vi "Driverstation.vi"   [LabVIEW 2012]
uses:
  Robot Global Data.vi
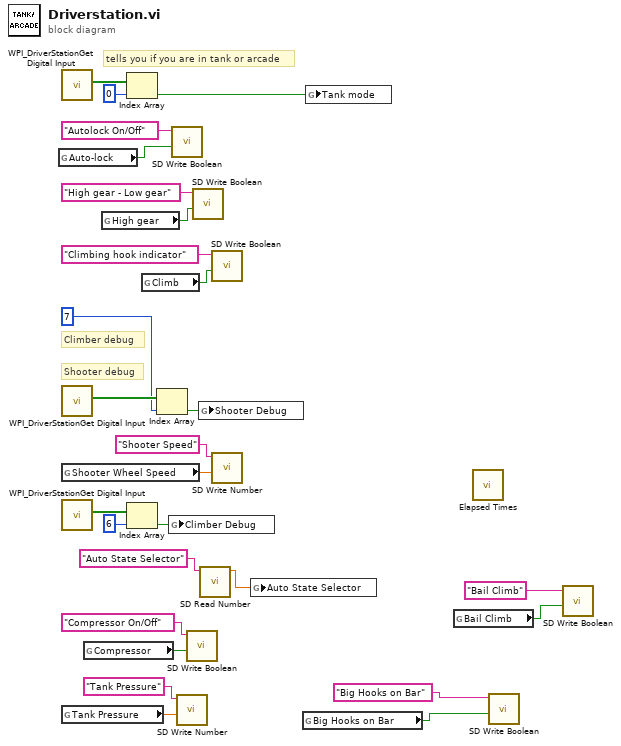
[diagram p0: block diagram]
diagram:
  # "Climber debug"
  # "Shooter debug"
  # "tells you if you are in tank or arcade"
  n1 = global read "Robot Global Data.vi" "Auto-lock"() -> (w5:bool)
  n2 = call <vilib>:"WPI_DriverStationGet Digital Input.vi"() -> ("Driver Station Digital Input (1-8)"=w27:bool[])  [unwired: 11 in]
  n3 = call <vilib>:"WPI_DriverStationGet Digital Input.vi"() -> ("Driver Station Digital Input (1-8)"=w24:bool[])  [unwired: 11 in]
  n4 = global read "Robot Global Data.vi" "Shooter Wheel Speed"() -> (w11:dbl)
  n5 = call <vilib>:"WPI_DriverStationGet Digital Input.vi"() -> ("Driver Station Digital Input (1-8)"=w20:bool[])  [unwired: 11 in]
  n6 = global read "Robot Global Data.vi" "Tank Pressure"() -> (w10:dbl)
  n7 = global read "Robot Global Data.vi" "Compressor"() -> (w9:bool)
  n8 = global read "Robot Global Data.vi" "High gear"() -> (w18:bool)
  n9 = Index Array(array=w27, index=0) -> (element=w25:bool)
  n10 = Index Array(array=w20, index=6) -> (element=w19:bool)
  n11 = global read "Robot Global Data.vi" "Climb"() -> (w15:bool)
  n12 = Index Array(array=w24, index=7) -> (element=w22:bool)
  n13 = global write "Robot Global Data.vi" "Climber Debug"(w19) -> ()
  n14 = call <vilib>:"SD Write Boolean.vi"("Boolean"=w5, "Name"="Autolock On/Off") -> ()  [unwired: 8 in, 2 out]
  n15 = call <vilib>:"SD Write Number.vi"("Numeric"=w10, "Name"="Tank Pressure") -> ()  [unwired: 8 in, 2 out]
  n16 = call <vilib>:"SD Write Boolean.vi"("Boolean"=w9, "Name"="Compressor On/Off") -> ()  [unwired: 8 in, 2 out]
  n17 = call <vilib>:"SD Write Boolean.vi"("Boolean"=w18, "Name"="High gear - Low gear") -> ()  [unwired: 8 in, 2 out]
  n18 = global write "Robot Global Data.vi" "Shooter Debug"(w22) -> ()
  n19 = call <vilib>:"SD Read Number.vi"("Name"="Auto State Selector") -> ("Numeric"=w6:dbl)  [unwired: 8 in, 2 out]
  n20 = call <vilib>:"SD Write Boolean.vi"("Boolean"=w15, "Name"="Climbing hook indicator") -> ()  [unwired: 8 in, 2 out]
  n21 = call <vilib>:"SD Write Number.vi"("Numeric"=w11, "Name"="Shooter Speed") -> ()  [unwired: 8 in, 2 out]
  n22 = global write "Robot Global Data.vi" "Auto State Selector"(w6) -> ()
  n23 = global read "Robot Global Data.vi" "Big Hooks on Bar"() -> (w3:bool)
  n24 = global write "Robot Global Data.vi" "Tank mode"(w25) -> ()
  n25 = global read "Robot Global Data.vi" "Bail Climb"() -> (w4:bool)
  n26 = call "Elapsed Times.vi"() -> ()  [unwired: 3 in, 1 out]
  n27 = call <vilib>:"SD Write Boolean.vi"("Boolean"=w3, "Name"="Big Hooks on Bar") -> ()  [unwired: 8 in, 2 out]
  n28 = call <vilib>:"SD Write Boolean.vi"("Boolean"=w4, "Name"="Bail Climb") -> ()  [unwired: 8 in, 2 out]
